vi "Msg Remain.vi"(10 "Remaining Elements":refnum<class "Msg.lvclass">[](array[class]), 11 "Self Actor in":refnum<class "Self Actor.lvclass">) -> ()   [LabVIEW 2021, in "AAM.lvlib" / "Self Actor.lvclass"]
uses:
  Self Actor.lvclass
  Msg/Msg.lvclass
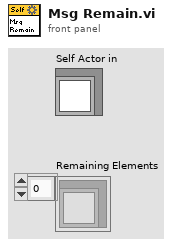
[diagram p1: front panel]
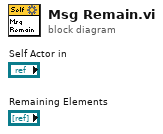
[diagram p0: block diagram]
diagram:
